vi "Turn to degrees.vi"(9 "Speed/Direction":dbl, 10 "Angle":dbl, 11 "RobotDriveDevRef in":T1) -> (3 "RobotDriveDevRef out":T1)   [LabVIEW 2015]
uses:
  <vilib>/Rock Robotics/WPI/RobotDrive/WPI_RobotDriveDevRef.ctl
  <vilib>/Rock Robotics/WPI/MotorControl/WPI_MotorControlDeviceRef.ctl
  <vilib>/Rock Robotics/WPI/MotorControl/WPI_MotorControlType.ctl
  <vilib>/Rock Robotics/SystemInterfaces/DIO/FPGA_DIOPWMChannel.ctl
  <vilib>/Rock Robotics/WPI/PWM/WPI_PWMDeadband.ctl
  <vilib>/Rock Robotics/WPI/CAN/Jaguar/SubVIs/WPI_CANJaguar_ControlMode.ctl
  <vilib>/Rock Robotics/WPI/CAN/TalonSRX/WPI_CANTalonSRX_APIControlMode.ctl
  <vilib>/Rock Robotics/WPI/RobotDrive/WPI_RobotDriveArcadeDrive_Standard(NoSaturation).vi
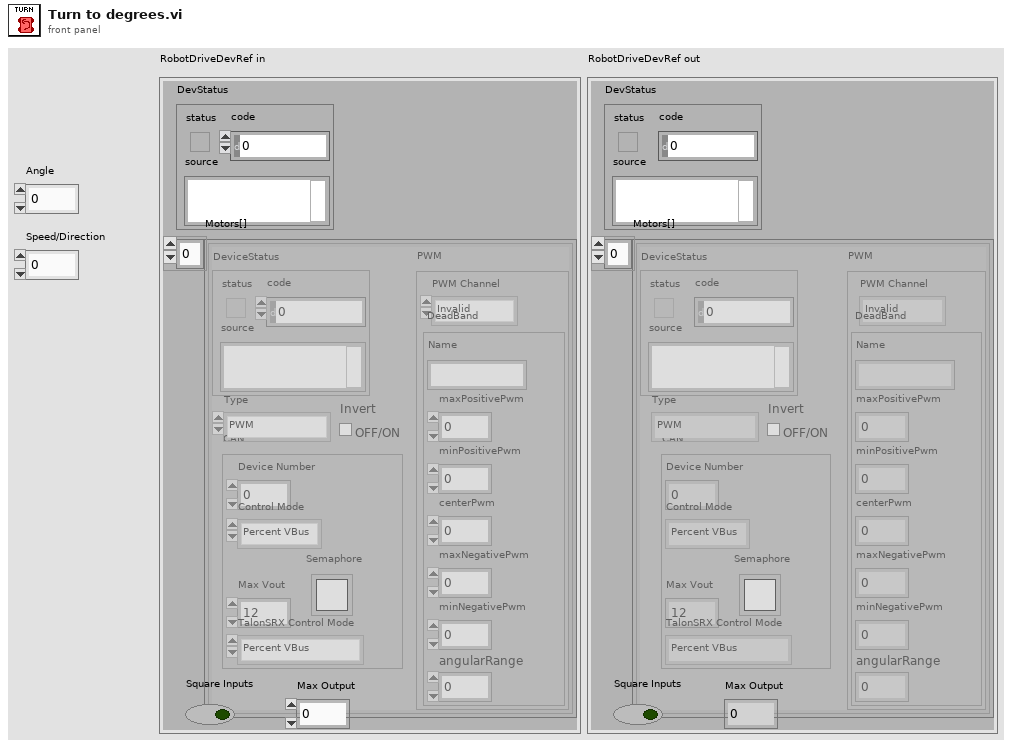
[diagram p1: front panel]
types:
  T1 = typedef "WPI_RobotDriveDevRef.ctl" = cluster{"DevStatus":errorcluster, "Motors[]":T2[], "Square Inputs":bool, "Max Output":dbl}
  T2 = typedef "WPI_MotorControlDeviceRef.ctl" = cluster{"DeviceStatus":errorcluster, "Type":T3, "PWM":cluster{"PWM Channel":T4, "DeadBand":T5}, "CAN":cluster{"Device Number":u8, "Control Mode":T6, "Semaphore":T7, "Max Vout":dbl, "TalonSRX Control Mode":T8}, "Invert":bool}
  T3 = typedef "WPI_MotorControlType.ctl" = enum16{"PWM", "CAN", "CANTalonSRX"}
  T4 = typedef "FPGA_DIOPWMChannel.ctl" = enum8{"PWM 0", "PWM 1", "PWM 2", "PWM 3", "PWM 4", "PWM 5", "PWM 6", "PWM 7", "PWM 8", "PWM 9", "PWM MXP 0", "PWM MXP 1", "PWM MXP 2", "PWM MXP 3", "PWM MXP 4", "PWM MXP 5", "PWM MXP 6", "PWM MXP 7", "PWM MXP 8", "PWM MXP 9", "Invalid"}
  T5 = typedef "WPI_PWMDeadband.ctl" = cluster{"Name":string, "maxPositivePwm":i32, "minPositivePwm":i32, "centerPwm":i32, "maxNegativePwm":i32, "minNegativePwm":i32, "angularRange":u16}
  T6 = typedef "WPI_CANJaguar_ControlMode.ctl" = enum8{"Percent VBus", "Current", "Speed", "Position", "Voltage"}
  T7 = typedef "Semaphore RefNum" = refnum<k1>
  T8 = typedef "WPI_CANTalonSRX_APIControlMode.ctl" = enum8{"Percent VBus", "Speed", "Position", "Slave", "Unchanged / Invalid", "Voltage Compensation", "Current", "Motion Profile"}
  T9 = typedef "WPI_GyroDevRef.ctl" = cluster{"DevStatus":errorcluster, "Analog Channel":T10, "Offset":dbl, "Gain (VoltsPerDegree/Second)":dbl, "Gyro Type":enum16{"Analog", "XRS450"}, "Handle":i32, "SPI Bus":T11, "Device Found":bool, "Sample Rate":dbl, "Calibrate On Open":bool}
  T10 = typedef "FPGA_AIChannel.ctl" = enum8{"AI 0", "AI 1", "AI 2", "AI 3", "AI MXP 0", "AI MXP 1", "AI MXP 2", "AI MXP 3", "Invalid"}
  T11 = typedef "spi_bus.ctl" = enum16{"SPI On-Board, CS0", "SPI On-Board, CS1", "SPI On-Board, CS2", "SPI On-Board, CS3", "SPI MXP", "Invalid"}
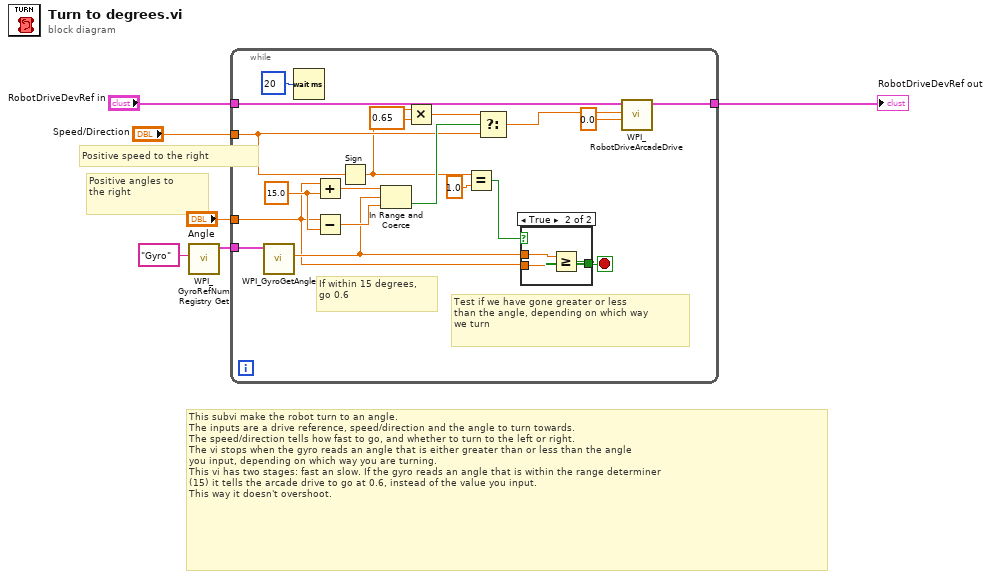
[diagram p0: block diagram]
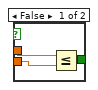
[diagram p2: hidden frame]
diagram:
  # "Positive speed to the right"
  # "Positive angles to\nthe right"
  # "This subvi make the robot turn to an angle.\nThe inputs are a drive reference, speed/direction and the angle to turn towards.\nThe speed/direction tells how fast to go, and whether to turn to the left or right.\nThe vi stops when the gyro reads an angle that is either greater than or less than the angle\nyou input, depending on which way you are turning.\nThis vi has two stages: fast an slow. If the gyro reads an angle that is within the range determiner\n(15) it tells the arcade drive to go at 0.6, instead of the value you input.\nThis way it doesn't overshoot."
  n1 = call <vilib>:"WPI_GyroRefNum Registry Get.vi"("refnum name"="Gyro") -> ("GyroDevRef"=w3:T9)  [unwired: 9 in, 1 out]
  n2 = while {
    tunnel: [w25] -> w6
    tunnel: "RobotDriveDevRef in" -> [w23]
    tunnel: w3 -> [w20]
    tunnel: "Angle" -> [w9]
    tunnel: "Speed/Direction" -> [w12]
    stop <- w8 stop-if-true
    w18 = 15.0
    # "If within 15 degrees,\ngo 0.6"
    # "Test if we have gone greater or less\nthan the angle, depending on which way\nwe turn"
    n3 = call <vilib>:"WPI_GyroGetAngle.vi"("GyroDevRef"=w20) -> ("Angle"=w14:dbl)  [unwired: 6 in, 4 out]
    n4 = Wait (ms)(milliseconds to wait=u32 20) -> ()  [unwired: 1 out]
    n5 = Add(x=w9, y=w18) -> (x+y=w16:dbl)
    n6 = Subtract(x=w9, y=w18) -> (x-y=w17:dbl)
    n7 = Sign(1:w12) -> (0:w10:dbl)
    n8 = In Range and Coerce(upper limit=w16, x=w14, lower limit=w17) -> (In Range?=w19:bool)  [unwired: 1 out]
    n9 = Multiply(x=0.65 ("t"), y=w10) -> (x*y=w11:dbl)
    n10 = Equal?(x=w10, y=1.0) -> (x = y?=w7:bool)
    n11 = Select(t=w11, s=w19, f=w12) -> (s? t:f=w15:dbl)
    n12 = case shown="True" w7 {
      tunnel: [w28 w31] -> w8
      tunnel: w14 -> [w26 w30]
      tunnel: w9 -> [w27 w29]
      frame False {
        n13 = Less Or Equal?(x=w26, y=w27) -> (x <= y?=w28:bool)
      }
      frame True {
        n14 = Greater Or Equal?(x=w30, y=w29) -> (x >= y?=w31:bool)
      }
    }
    n15 = call-poly <vilib>:"WPI_RobotDriveArcadeDrive.vi"("Y axis value"=0.0, "X axis value"=w15, "RobotDriveDevRef"=w23) -> ("RobotDriveDevRef"=w25:T1)  [unwired: 6 in, 2 out]
  }
  "RobotDriveDevRef out" <- w6
